vi "getTopicSubscriptions.vi"(8 "error in (no error)":errorcluster, 11 "UNSUBSCRIBE in":refnum<class "UNSUBSCRIBE.lvclass">) -> (0 "error out":errorcluster, 2 "Topic Subscriptions":string[](array[string]), 3 "UNSUBSCRIBE out":refnum<class "UNSUBSCRIBE.lvclass">)   [LabVIEW 2013, in "MQTT_Control_Packets.lvlib" / "UNSUBSCRIBE.lvclass"]
uses:
  UNSUBSCRIBE.lvclass
  ControlPacket/ControlPacket.lvclass/ControlPacket.ctl
  ControlPacket/ControlPacket.lvclass
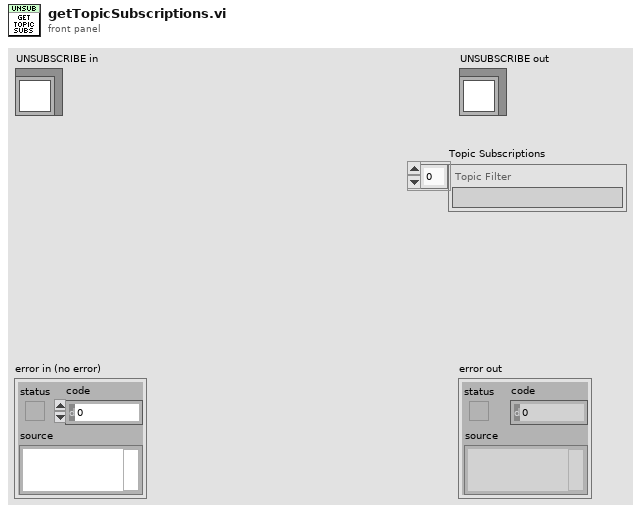
[diagram p1: front panel]
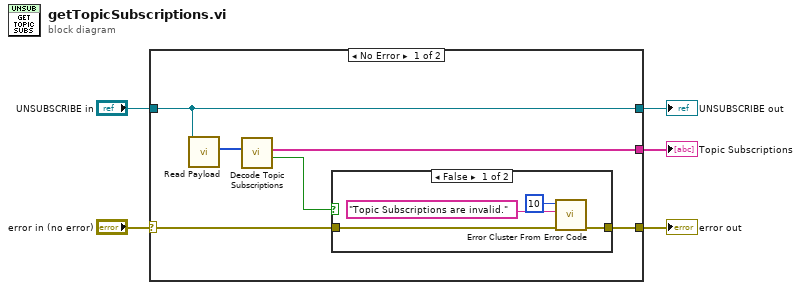
[diagram p0: block diagram]
diagram:
  n1 = case shown="No Error" "error in (no error)" {
    selector: "error in (no error)" -> [w7 w18]
    tunnel: [w6 w18] -> w4
    tunnel: [w11 w17] -> w2
    tunnel: "UNSUBSCRIBE in" -> [w11 w17]
    tunnel: [w9 _] -> w1
    frame No Error {
      n2 = call "Read Payload.vi"("ControlPacket in"=w11) -> ("Payload"=w10:u8[])  [unwired: 9 in, 1 out]
      n3 = call "Decode Topic Subscriptions.vi"("Payload"=w10) -> ("Valid?"=w8:bool, "Topic Subscriptions"=w9:string[])  [unwired: 9 in]
      n4 = case shown="False" w8 {
        tunnel: w7 -> [w15 w16]
        tunnel: [w12 w16] -> w6
        frame False {
          n5 = call <vilib>:"Error Cluster From Error Code.vi"("error in (no error)"=w15, "error message (\"\")"="Topic Subscriptions are invalid." ("error source (\" \")"), "error code (0)"=10 ("error code (no error:0)")) -> ("error out"=w12:errorcluster)  [unwired: 6 in]
        }
        frame True {
        }
      }
    }
    frame Error {
    }
  }
  "error out" <- w4
  "UNSUBSCRIBE out" <- w2
  "Topic Subscriptions" <- w1
